vi "Open_Comm.vi"(8 "error in (no error)":errorcluster caption="entrée d'erreur (pas d'erreur)", 11 "Class Shielding_ Box en entrée":refnum<class "Class Shielding_ Box JC-PB3044.lvclass">) -> (0 "error out":errorcluster caption="sortie d'erreur", 3 "Class Shielding_ Box en sortie":refnum<class "Class Shielding_ Box JC-PB3044.lvclass">)   [LabVIEW 2020, in "Library Instrument & Equipement.lvlib" / "Library Shielding box.lvlib" / "Class Shielding_ Box JC-PB3044.lvclass"]
uses:
  Class Shielding_ Box JC-PB3044.lvclass
  C:/Users/ngarcin/OneDrive - Altyor/Standard TB/Class/Shielding box/Class Shielding box (Default)/Class Shielding_ Box (Default).lvclass
  <vilib>/Instr/_visa.llb/VISA Configure Serial Port (Instr).vi
  Class Shielding_ Box JC-PB3044.lvclass/Class Shielding_ Box JC-PB3044.ctl
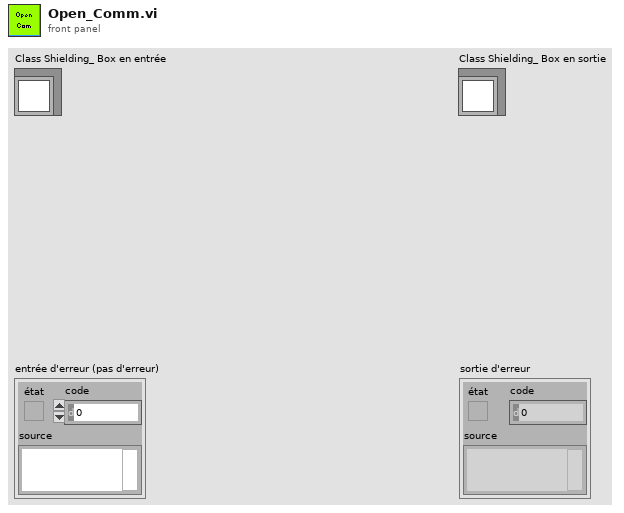
[diagram p1: front panel]
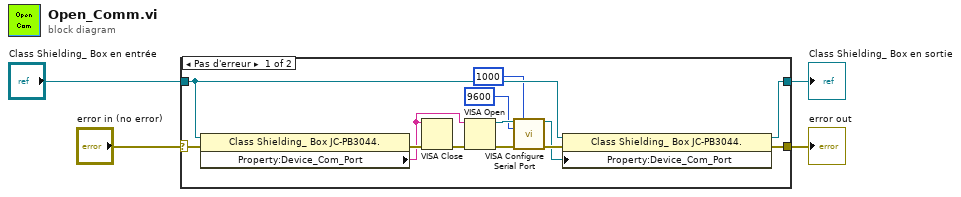
[diagram p0: block diagram]
diagram:
  n1 = case shown="Pas d'erreur" "error in (no error)" {
    selector: "error in (no error)" -> [w11 w19]
    tunnel: [w6 w19] -> w3
    tunnel: [w7 w18] -> w1
    tunnel: "Class Shielding_ Box en entrée" -> [w10 w18]
    frame No Error {
      n2 = property class="Class Shielding_ Box JC-PB3044."(reference=w10, error in=w11) -> (error out=w13:errorcluster, "Property:Device_Com_Port"=w12:string)  [unwired: 1 out]
      n3 = VISA Close(VISA resource name=w12, error in (no error)=w13) -> (error out=w14:errorcluster)
      n4 = VISA Open(error in (no error)=w14, VISA resource name=w12) -> (VISA resource name=w17:refnum<visa-resource-name>, error out=w15:errorcluster)  [unwired: 3 in]
      n5 = call-poly "VISA Configure Serial Port"("VISA resource name"=w17, "timeout (10sec)"=u32 1000, "baud rate (9600)"=u32 9600, "error in (no error)"=w15) -> ("VISA resource name out"=w8:refnum<visa-resource-name>, "error out"=w9:errorcluster)  [unwired: 10 in]
      n6 = property class="Class Shielding_ Box JC-PB3044."(reference=w10, error in=w9, "Property:Device_Com_Port"=w8) -> (reference out=w7:refnum<class "Class Shielding_ Box JC-PB3044.lvclass">, error out=w6:errorcluster)
    }
    frame Error {
    }
  }
  "error out" <- w3
  "Class Shielding_ Box en sortie" <- w1
